vi "readSGL.vi"(8 "error in (no error)":errorcluster, 11 "ModbusBuffer in":refnum<class "ModbusBuffer.lvclass">) -> (0 "error out":errorcluster, 2 "Output":sgl, 3 "ModbusBuffer out":refnum<class "ModbusBuffer.lvclass">)   [LabVIEW 2016, in "RTModbus.lvlib" / "ModbusBuffer.lvclass"]
uses:
  ModbusBuffer.lvclass
  ModbusBuffer.lvclass/ModbusBuffer.ctl
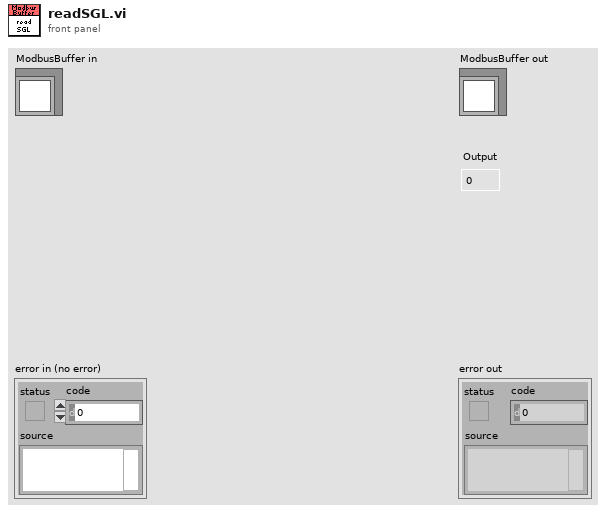
[diagram p1: front panel]
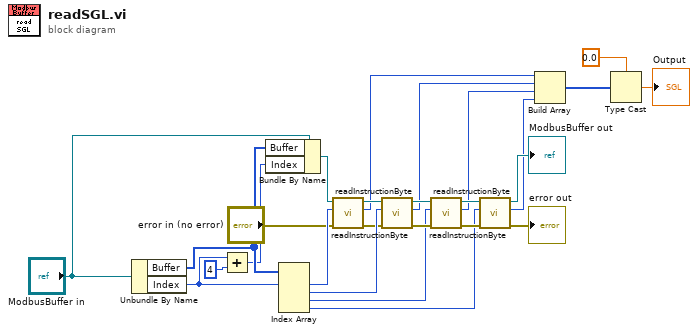
[diagram p0: block diagram]
diagram:
  n1 = Unbundle By Name("ModbusBuffer in") -> ("Buffer"=w25:u16[], "Index"=w21:i32)
  n2 = Add(x=w21, y=4) -> (x+y=w19:i32)
  n3 = Bundle By Name(cluster="ModbusBuffer in", "Buffer"=w25, "Index"=w19) -> (w23:refnum<class "ModbusBuffer.lvclass">)
  n4 = Index Array(array=w25, index #1=w21) -> (element #1=w24:u16, element #2=w17:u16, element #3=w11:u16, element #4=w10:u16)  [unwired: 3 in]
  n5 = call "readInstructionByte.vi"("error in (no error)"="error in (no error)", "Instruction"=w24, "ModbusBuffer in"=w23) -> ("error out"=w16:errorcluster, "Output"=w4:u8, "ModbusBuffer out"=w18:refnum<class "ModbusBuffer.lvclass">)  [unwired: 6 in]
  n6 = call "readInstructionByte.vi"("error in (no error)"=w16, "Instruction"=w17, "ModbusBuffer in"=w18) -> ("error out"=w13:errorcluster, "Output"=w3:u8, "ModbusBuffer out"=w15:refnum<class "ModbusBuffer.lvclass">)  [unwired: 6 in]
  n7 = call "readInstructionByte.vi"("error in (no error)"=w13, "Instruction"=w11, "ModbusBuffer in"=w15) -> ("error out"=w12:errorcluster, "Output"=w2:u8, "ModbusBuffer out"=w14:refnum<class "ModbusBuffer.lvclass">)  [unwired: 6 in]
  n8 = call "readInstructionByte.vi"("error in (no error)"=w12, "Instruction"=w10, "ModbusBuffer in"=w14) -> ("error out"=→"error out":errorcluster, "Output"=w1:u8, "ModbusBuffer out"=→"ModbusBuffer out":refnum<class "ModbusBuffer.lvclass">)  [unwired: 6 in]
  n9 = Build Array(w4, w3, w2, w1) -> (w9:u8[])
  n10 = Type Cast(type=sgl 0.0, x=w9) -> (*(type *) &x=→"Output":sgl)
